vi "Stop Image.vi"(10 "Image Array In":i32[](array[numeric]), 11 "Pixel Array In":i32[](array[numeric])) -> (3 "Pixel Array Out":i32[](array[numeric]))   [LabVIEW 2019]
doc: "Removes the fire image source by randomly decreasing its intensity until it is removed completely. Repeated calls to Do Fire.vi will then burn up the remainder of the fire."
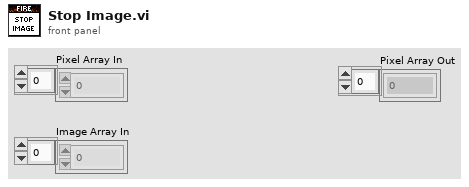
[diagram p1: front panel]
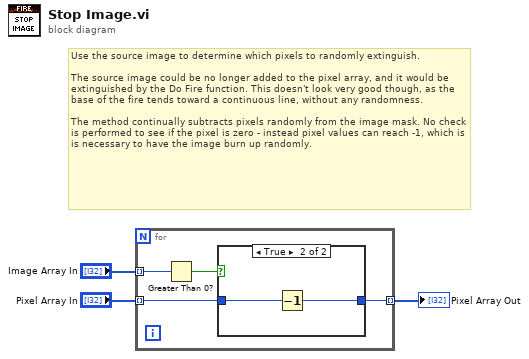
[diagram p0: block diagram]
diagram:
  # "Use the source image to determine which pixels to randomly extinguish.\n\nThe source image could be no longer added to the pixel array, and it would be extinguished by the Do Fire function. This doesn't look very good though, as the base of the fire tends toward a continuous line, without any randomness.\n\nThe method continually subtracts pixels randomly from the image mask. No check is performed to see if the pixel is zero - instead pixel values can reach -1, which is is necessary to have the image burn up randomly."
  n1 = for {
    tunnel: "Pixel Array In" -> [w5] mode=indexing
    tunnel: "Image Array In" -> [w6] mode=indexing
    tunnel: [w7] -> w1 mode=indexing
    n2 = Greater Than 0?(x=w6) -> (x > 0?=w4:bool)
    n3 = case shown="True" w4 {
      tunnel: w5 -> [w8 w10]
      tunnel: [w8 w9] -> w7
      frame False {
      }
      frame True {
        n4 = Decrement(x=w10) -> (x-1=w9:i32)
      }
    }
  }
  "Pixel Array Out" <- w1
